vi "test.top.level.vi"() -> ()   [LabVIEW 2021]
uses:
  <vilib>/rvi/interface/RandomDataEmulation/nirviRandomDataOpen.vi
  <vilib>/rvi/interface/common/niFpgaCacheSessionInfoDynamic.vi
  <vilib>/FPGAPlugInAG/Dynamic/niLvFpga_Close_Dynamic.vi
  <vilib>/rvi/interface/nirviOpenFPGA/nirviOpenFPGA.xnode
  fpga/keccak.fpga.top.vi
  <vilib>/rvi/interface/nirviCloseFPGA/nirviCloseFPGA.xnode
panel:
  in  "Start.Index":i32
  out "All 512 FPGA Pass?":bool=TRUE
  out "All 256 FPGA Pass?":bool=TRUE
  out "Host - FPGA Results Details":T1(array[cluster])
  in  "Test Cases":i32=1
  out "FPGA 256\nMatches?":bool=TRUE
  out "FPGA 512 Matches?":bool=TRUE
  out "Fpga.Results (256)":u64[](array[numeric]) format="%.0x"
  out "Fpga.Results (512)":u64[](array[numeric]) format="%.0x"
  in  "Enable FPGA\nTests?":bool
  out "Data.in.U64":u64[](array[numeric]) format="%.0x"
  out "error out":errorcluster
  in  "error in":errorcluster
  out "All 512 Host Pass?":bool=TRUE
  out "All 256 Host Pass?":bool=TRUE
  out "Data.In.U8":u8[](array[numeric])=[65, 115, 32, 69, 115, 116, 104, 97, 32, 115, 116, 105, 114, 114, 101, 100, 32, 116, 104, 101, 32, 116, 104, 105, 99, 107, 32, 106, 97, 109, 32, 104, 101, 32, 116, 104, 111, 117, 103, 104, 116, 32, 84, 119, 111, 32, 84, 104, 111, 117, 103, 104, 116, 115, 32, 97, 110, 100, 32, 116, 104, 101, 32, 84, 119, 111, 32, 84, 104, 111, 117, 103, 104, 116, 115, 32, 104, 101, 32, 116, 104, 111, 117, 103, 104, 116, 32, 119, 101, 114, 101, 32, 116, 104, 101, 115, 101, 58, 32, 97, 41, 32, 65, 110, 121, 116, 104, 105, 110, 103, 32, 99, 97, 110, 32, 104, 97, 112, 112, 101, 110, 32, 116, 111, 32, 97, 110, 121, 111, 110, 101, 46, 32, 97, 110, 100, 32, 98, 41, 32, 73, 116, 32, 105, 115, 32, 98, 101, 115, 116, 32, 116, 111, 32, 98, 101, 32, 112, 114, 101, 112, 97, 114, 101, 100, 46] format="%.0x"
  out "512 matches?":bool=TRUE
  out "Final.State 512":u64[](array[numeric])=[13301219531156492385, 11127854853417562052, 524277580094970210, 1540142370391429374, 12412996341010901443, 3598767773402858399, 924216014969962459, 18423737124033093736, 9041965587285169724, 11946436709797590620, 9598377346200053498, 15609136642136624313, 13839031544369048776, 16785932279372823442, 18077763469661243185, 6037779733261654142, 5492308379086555739, 2813253888995526086, 3560799791317313623, 11061351188809493633, 14966076467780343448, 9073521057931985780, 7504373216799846216, 2649547696616143726, 14741899879960970636] format="%.0x"
  out "256 matches?":bool=TRUE
  out "Final.State 256":u64[](array[numeric])=[11676268880411235193, 13451318828874210226, 4095211424469938024, 15068679232636183629, 7753535997560901512, 5388403742991398886, 18434487315843317224, 9964010514430008916, 15544274158139793918, 17249301923950297777, 11191994372900048372, 9929105044359600294, 9415787041053954757, 3504658296181967959, 5125580019117546070, 12884011986622445834, 10134502102761320058, 17607174279953371043, 17308940434400663160, 5579560056542968276, 9133654056512198443, 18102584358251476685, 2528813078336136997, 14545830983934253368, 1290234347948013036] format="%.0x"
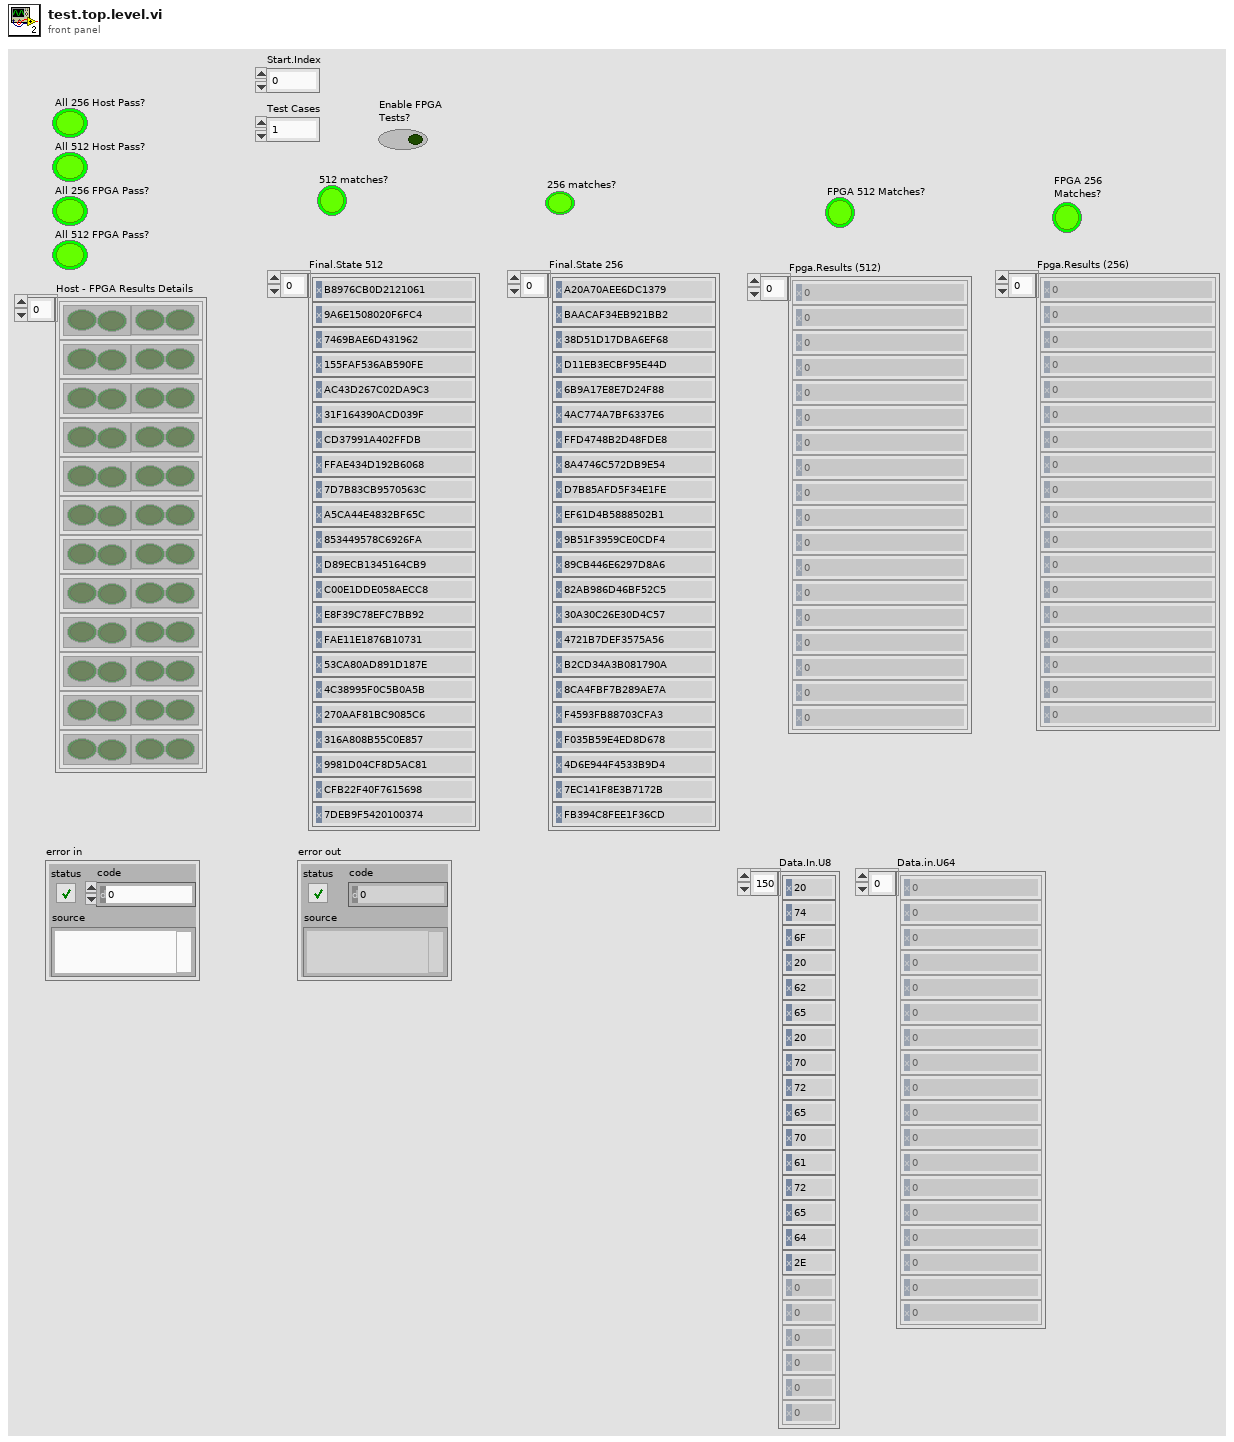
[diagram p1: front panel]
types:
  T1 = cluster{cluster{bool, bool}, cluster{bool, bool}}[]
  T2 = typedef "Test.Case.type.ctl" = cluster{"input_size":i32, "expected_hash256":string, "expected_hash512":string}
  T3 = cluster{"input_size":i32, "Bits.in":u32, "Array":u64[]}
  T4 = cluster{cluster{bool, bool}, cluster{bool, bool}}
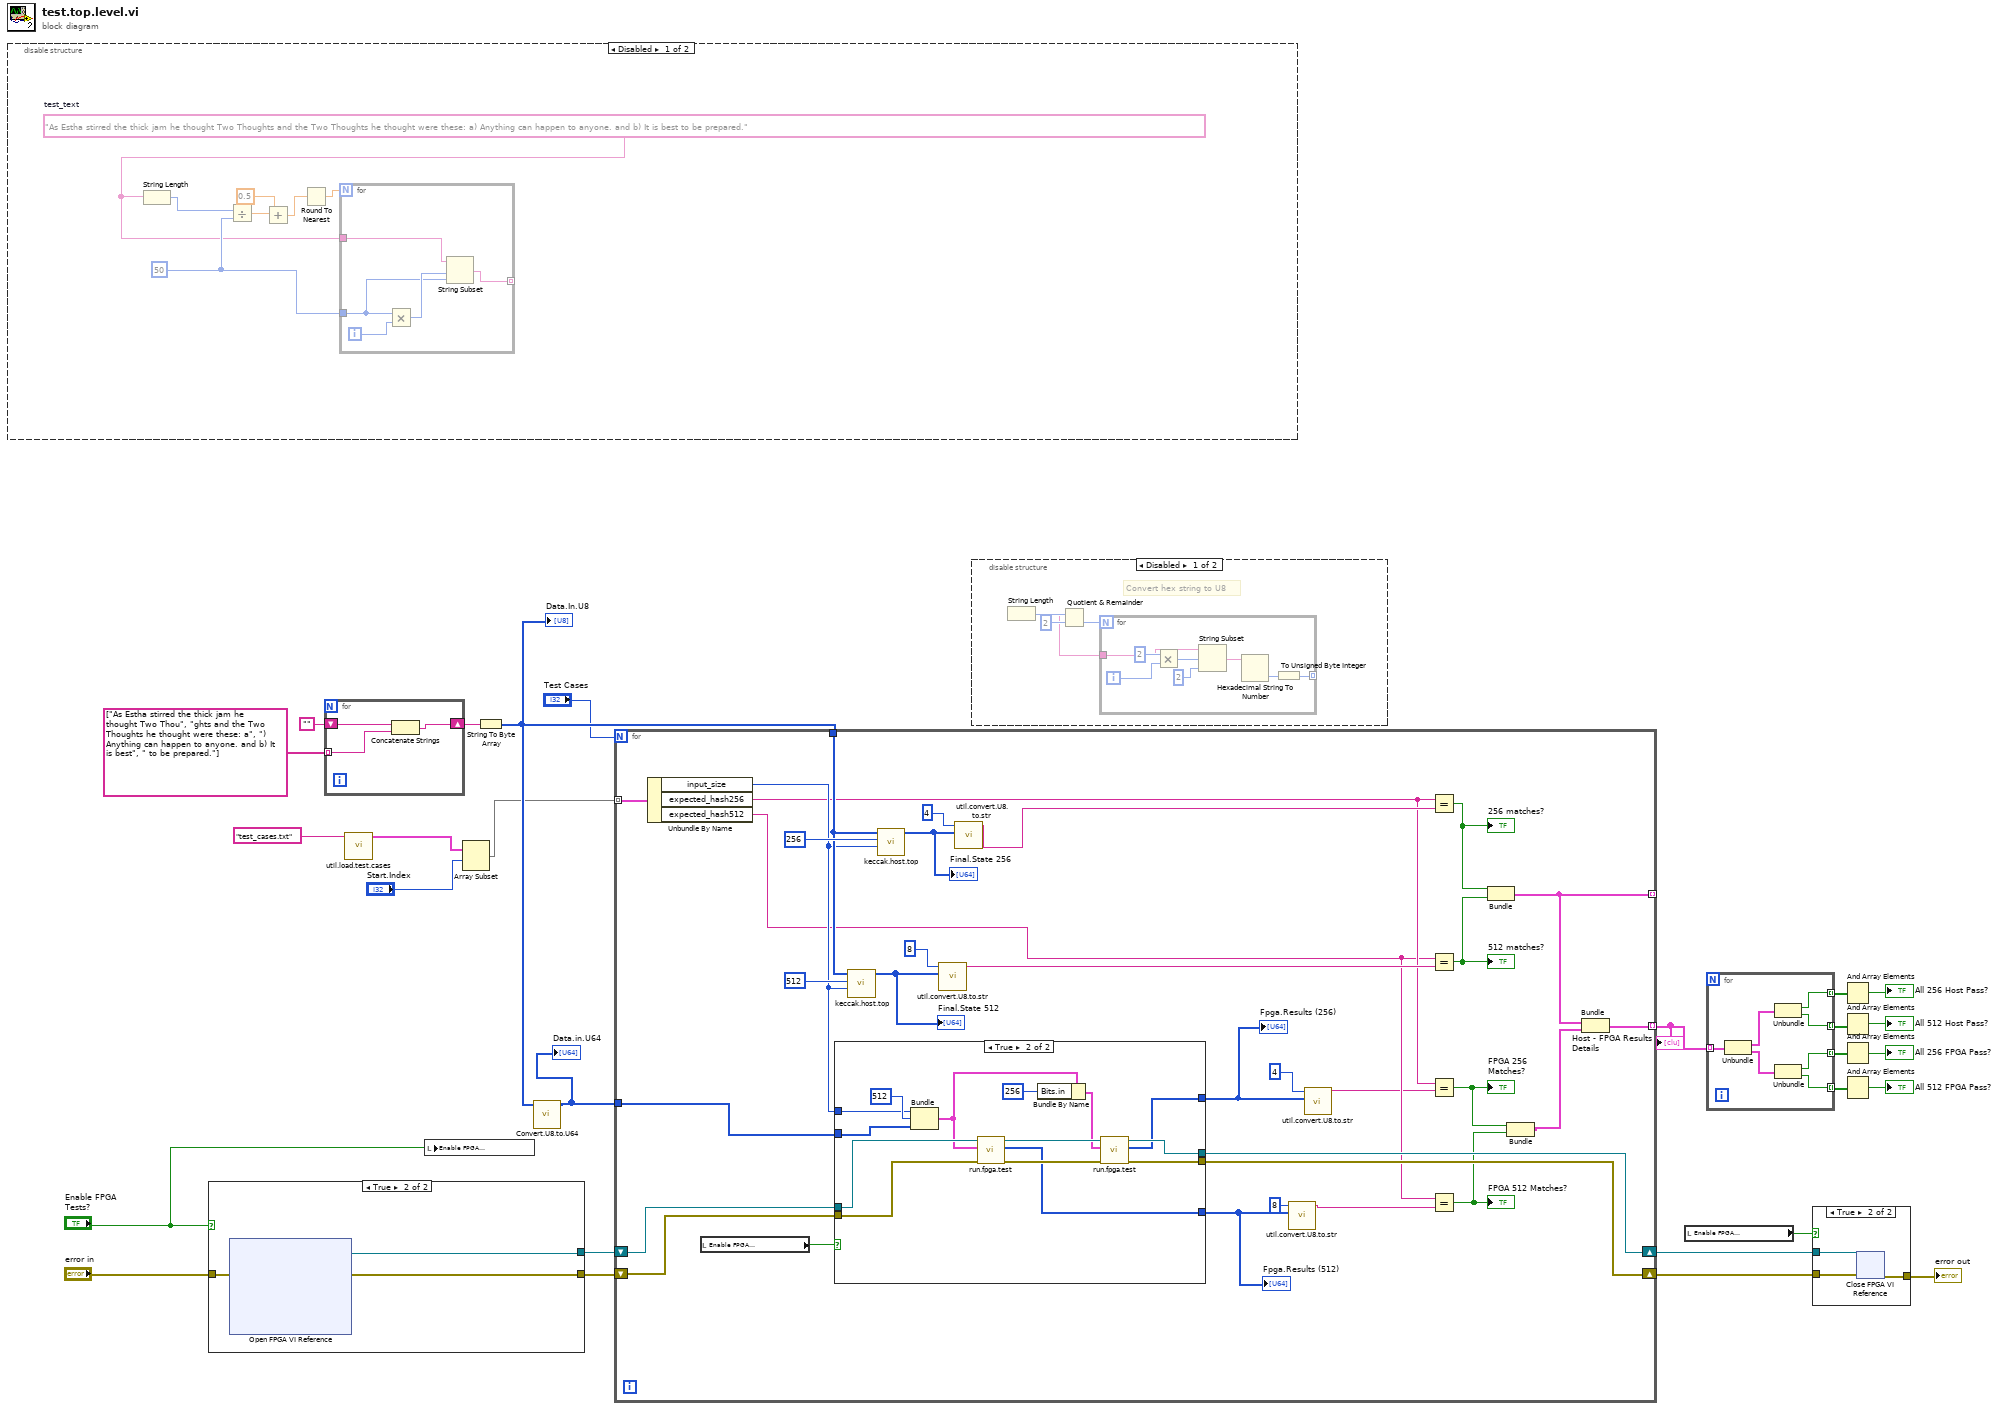
[diagram p0: block diagram]
diagram:
  n1 = disable-structure shown="Disabled" {
    frame Disabled {
      w33 = 50 ("y")
      w28 = "As Estha stirred the thick jam he thought Two Thoughts and the Two Thoughts he thought were these: a) Anything can happen to anyone. and b) It is best to be prepared."  # test_text
      n2 = String Length(string=w28) -> (length=w34:i32)
      n3 = Divide(x=w34, y=w33) -> (x/y=w32:dbl)
      n4 = Add(x=w32, y=0.5) -> (x+y=w30:dbl)
      n5 = Round To Nearest(number=w30) -> (nearest integer value=w29:dbl)
      n6 = for {
        N: w29 -> [_]
        tunnel: w33 -> [w37]
        tunnel: w28 -> [w36]
        tunnel: [w35] -> _ mode=indexing
        i -> [w38]
        n7 = Multiply(x=w37, y=w38) -> (x*y=w39:i32)
        n8 = String Subset(string=w36, offset (0)=w39, length (rest)=w37) -> (substring=w35:string)
      }
    }
    frame Enabled {
    }
  }
  n9 = case shown="True" "Enable FPGA\nTests?" {
    tunnel: "error in" -> [w40 w43]
    tunnel: [w40 w42] -> w23
    tunnel: [_ w41] -> w22
    frame False {
    }
    frame True {
      n10 = xnode "Open FPGA VI Reference"("error in"=w43) -> ("FPGA VI Reference Out"=w41:refnum<k20>, "error out"=w42:errorcluster)  [unwired: 1 in]
    }
  }
  n11 = for {
    tunnel: string[] ["As Estha stirred the thick jam he thought Two Thou", "ghts and the Two Thoughts he thought were these: a", ") Anything can happen to anyone. and b) It is best", " to be prepared."] ("Array 2") -> [w45] mode=indexing
    shift-right: [w44] -> w15
    shift-left: "" -> [w46]
    n12 = Concatenate Strings(w46, w45) -> (w44:string)
  }
  n13 = call "util.load.test.cases.vi"("String"="test_cases.txt") -> ("Array"=w3:T2[])  [unwired: 10 in]
  n14 = local write "Enable FPGA\nTests?"("Enable FPGA\nTests?") -> ()
  n15 = Array Subset(array=w3, index="Start.Index") -> (w2:T2[])  [unwired: 1 in]
  n16 = String To Byte Array(string=w15) -> (unsigned byte array=w24:u8[])
  "Data.In.U8" <- w24
  n17 = call "Convert.U8.to.U64.vi"("unsigned byte array"=w24) -> ("Array"=w13:u64[])  [unwired: 9 in, 1 out]
  "Data.in.U64" <- w13
  n18 = for {
    N: "Test Cases" -> [_]
    tunnel: w2 -> [w73] mode=indexing
    tunnel: w24 -> [w72]
    tunnel: [w49] -> _ mode=indexing
    shift-right: [w65] -> w18
    shift-left: w22 -> [w69]
    shift-right: [w64] -> w17
    shift-left: w23 -> [w67]
    tunnel: w13 -> [w66]
    tunnel: [w47] -> w12 mode=indexing
    n19 = Unbundle By Name(w73) -> ("input_size"=w63:i32, "expected_hash256"=w55:string, "expected_hash512"=w54:string)
    n20 = local read "Enable FPGA\nTests?"() -> (w68:bool)
    n21 = case shown="True" w68 {
      tunnel: w69 -> [w80 w94]
      tunnel: w67 -> [w79 w93]
      tunnel: w63 -> [_ w91]
      tunnel: w66 -> [_ w90]
      tunnel: [w80 w85] -> w65
      tunnel: [w79 w87] -> w64
      tunnel: [_ w82] -> w61
      tunnel: [_ w81] -> w60
      frame False {
      }
      frame True {
        n22 = Bundle("input_size"=w91, "Bits.in"=u32 512, "Array"=w90) -> (w89:T3)  [unwired: 1 in]
        n23 = call "run.fpga.test.vi"("error in (no error)"=w93, "Test.Parms"=w89, "Refnum in"=w94) -> ("error out"=w83:errorcluster, "Fpga\nData.out"=w81:u64[], "Refnum out"=w86:refnum<k20>)  [unwired: 6 in]
        n24 = Bundle By Name(cluster=w89, "Bits.in"=u32 256) -> (w84:T3)
        n25 = call "run.fpga.test.vi"("error in (no error)"=w83, "Test.Parms"=w84, "Refnum in"=w86) -> ("error out"=w87:errorcluster, "Fpga\nData.out"=w82:u64[], "Refnum out"=w85:refnum<k20>)  [unwired: 6 in]
      }
    }
    "Fpga.Results (256)" <- w61
    "Fpga.Results (512)" <- w60
    n26 = call "keccak.host.top.vi"("size"=w63, "Bits.in"=512, "Data.in"=w72) -> ("Final.State"=w77:u64[])  [unwired: 8 in]
    "Final.State 512" <- w77
    n27 = call "keccak.host.top.vi"("size"=w63, "Bits.in"=256, "Data.in"=w72) -> ("Final.State"=w57:u64[])  [unwired: 8 in]
    "Final.State 256" <- w57
    n28 = call "util.convert.U8.to.str.vi"("Final.State"=w77, "Numeric"=8) -> ("String"=w74:string)  [unwired: 9 in]
    n29 = call "util.convert.U8.to.str.vi"("Final.State"=w57, "Numeric"=4) -> ("String"=w56:string)  [unwired: 9 in]
    n30 = call "util.convert.U8.to.str.vi"("Final.State"=w60, "Numeric"=8) -> ("String"=w53:string)  [unwired: 9 in]
    n31 = call "util.convert.U8.to.str.vi"("Final.State"=w61, "Numeric"=4) -> ("String"=w52:string)  [unwired: 9 in]
    n32 = Equal?(x=w55, y=w56) -> (x = y?=w71:bool)
    "256 matches?" <- w71
    n33 = Equal?(x=w54, y=w74) -> (x = y?=w70:bool)
    "512 matches?" <- w70
    n34 = Equal?(x=w55, y=w52) -> (x = y?=w51:bool)
    "FPGA 256\nMatches?" <- w51
    n35 = Equal?(x=w54, y=w53) -> (x = y?=w50:bool)
    "FPGA 512 Matches?" <- w50
    n36 = Bundle(w71, w70) -> (w49:cluster{bool, bool})  [unwired: 1 in]
    n37 = Bundle(w51, w50) -> (w48:cluster{bool, bool})  [unwired: 1 in]
    n38 = Bundle(w49, w48) -> (w47:T4)  [unwired: 1 in]
  }
  "Host - FPGA Results Details" <- w12
  n39 = disable-structure shown="Disabled" {
    frame Disabled {
      # "Convert hex string to U8"
      n40 = String Length() -> (string=w95:string, length=w98:i32)
      n41 = Quotient & Remainder(x=w98, y=2) -> (floor(x/y)=w96:i32)  [unwired: 1 out]
      n42 = for {
        N: w96 -> [_]
        tunnel: w95 -> [w102]
        tunnel: [w99] -> _ mode=indexing
        i -> [w106]
        n43 = Multiply(x=2, y=w106) -> (x*y=w105:i32)
        n44 = String Subset(string=w102, offset (0)=w105, length (rest)=2 ("length (rest)")) -> (substring=w101:string)
        n45 = Hexadecimal String To Number(string=w101) -> (number=w100:u32)  [unwired: 2 in, 1 out]
        n46 = To Unsigned Byte Integer(number=w100) -> (unsigned 8bit integer=w99:u8)
      }
    }
    frame Enabled {
    }
  }
  n47 = local read "Enable FPGA\nTests?"() -> (w19:bool)
  n48 = for {
    tunnel: w12 -> [w113] mode=indexing
    tunnel: [w110] -> w8 mode=indexing
    tunnel: [w109] -> w9 mode=indexing
    tunnel: [w108] -> w10 mode=indexing
    tunnel: [w107] -> w11 mode=indexing
    n49 = Unbundle(w113) -> (w111:cluster{bool, bool}, w112:cluster{bool, bool})
    n50 = Unbundle(w111) -> (w110:bool, w109:bool)
    n51 = Unbundle(w112) -> (w108:bool, w107:bool)
  }
  n52 = case shown="True" w19 {
    tunnel: [w114 w117] -> w25
    tunnel: w18 -> [_ w116]
    tunnel: w17 -> [w114 w115]
    frame False {
    }
    frame True {
      n53 = xnode "Close FPGA VI Reference"("FPGA VI Reference In"=w116, "error in"=w115) -> ("error out"=w117:errorcluster)
    }
  }
  "error out" <- w25
  n54 = And Array Elements(Boolean array=w8) -> (logical AND=→"All 256 Host Pass?":bool)
  n55 = And Array Elements(Boolean array=w9) -> (logical AND=→"All 512 Host Pass?":bool)
  n56 = And Array Elements(Boolean array=w10) -> (logical AND=→"All 256 FPGA Pass?":bool)
  n57 = And Array Elements(Boolean array=w11) -> (logical AND=→"All 512 FPGA Pass?":bool)
